vi "GetPicture.vi"() -> ()   [LabVIEW 2011]
panel:
  in  "GetPicture":bool
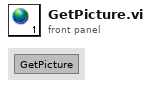
[diagram p1: front panel]
diagram:
